vi "Step ADD GND W Parameters.vi"(0 "VISA resource name":refnum<visa-resource-name>, 1 "Scanner Selection in (0)":i32, 2 "Internal scanner?":bool, 5 "GND Test Parameters in":T1={"Current (25 A)"=25.0, "Voltage (8 V)"=8.0, "Hi-Limit (100 mohm)"=100.0, "Lo-Limit (0 mohm)"=0.0, "Dwell (1 s)"=1.0, "Offset (0 mohm)"=0.0, "Auto Offset (OFF)"=FALSE} {"Offset (0 mohm)" format="%#.2f"; "Lo-Limit (0 mohm)" format="%#.2f"; "Hi-Limit (100 mohm)" format="%#.2f"}, 7 "Step Selection (1-200)":i32=1, 9 "Add Step":bool, 11 "error in (no error)":errorcluster) -> (4 "VISA resource name out":refnum<visa-resource-name>, 15 "error out":errorcluster)   [LabVIEW 2014]
doc: "Inserts a GND test with the User defined parameters into the assigned Step Selecton.\n\nIf Add step is set to Edit, it will replace the existing step. If it is set to Add it will insert the new step and increment all steps after the selected step by 1.\n\nSee specifications for Limits."
uses:
  <instrlib>/eec EST 300/eec EST 300.lvlib
  <instrlib>/EEC EST 300/Public/Configure/Steps/Low Level/GND Test Parameters.ctl
panel:
  # "Add"
  # "Edit"
  # "ON"
  # "OFF"
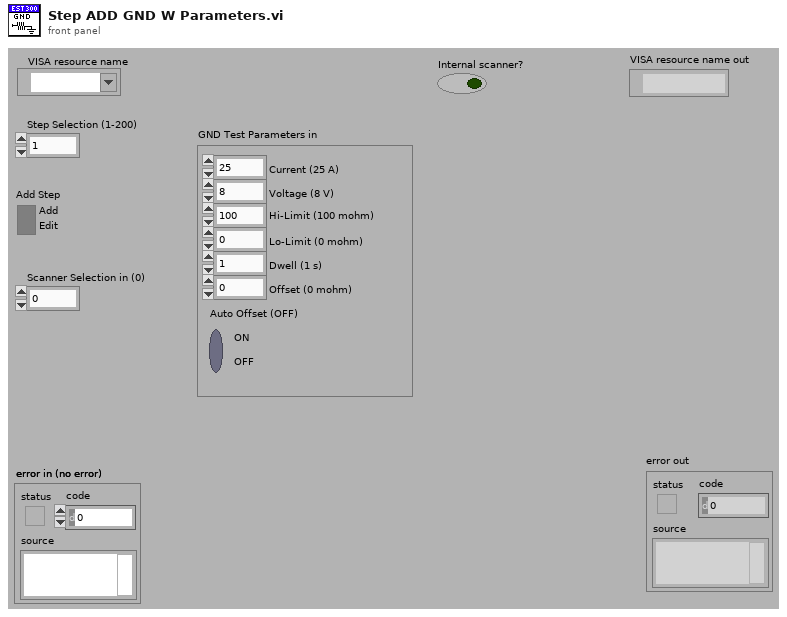
[diagram p1: front panel]
types:
  T1 = typedef "EEC EST 300.lvlib/GND Test Parameters.ctl" = cluster{"Current (25 A)":dbl, "Voltage (8 V)":dbl, "Hi-Limit (100 mohm)":dbl, "Lo-Limit (0 mohm)":dbl, "Dwell (1 s)":dbl, "Offset (0 mohm)":dbl, "Auto Offset (OFF)":bool}
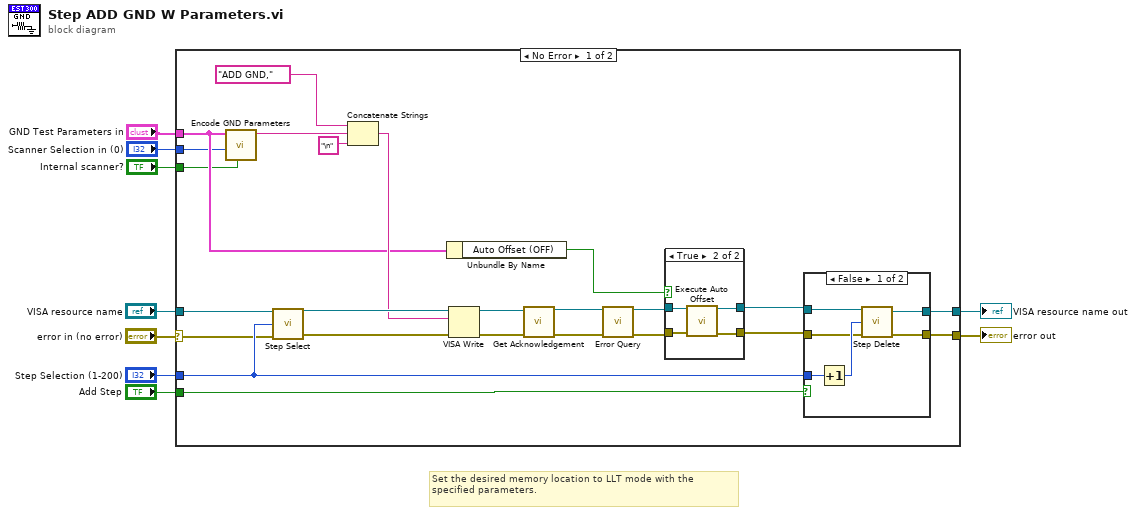
[diagram p0: block diagram]
diagram:
  # "Set the desired memory location to LLT mode with the specified parameters."
  n1 = case shown="No Error" "error in (no error)" {
    selector: "error in (no error)" -> [w22 w49]
    tunnel: [w31 w49] -> w8
    tunnel: [w30 w48] -> w6
    tunnel: "VISA resource name" -> [w23 w48]
    tunnel: "Step Selection (1-200)" -> [w24 _]
    tunnel: "Add Step" -> [w29 _]
    tunnel: "Internal scanner?" -> [w10 _]
    tunnel: "GND Test Parameters in" -> [w12 _]
    tunnel: "Scanner Selection in (0)" -> [w11 _]
    frame No Error {
      n2 = call <instrlib>:"Encode GND Parameters.vi"("scanner? (F:No)"=w10, "Scanner Selection in (0)"=w11, "GND Test Parameters in"=w12) -> ("ADD Parameters out"=w13:string)  [unwired: 6 in, 2 out]
      n3 = call <instrlib>:"Step Select.vi"("VISA resource name"=w23, "Step Number (1)"=w24, "error in (no error)"=w22) -> ("VISA resource name out"=w32:refnum<visa-resource-name>, "error out"=w33:errorcluster)  [unwired: 11 in]
      n4 = Concatenate Strings("ADD GND," ("string"), w13, "\n" ("string")) -> (w27:string)
      n5 = Unbundle By Name(w12) -> ("Auto Offset (OFF)"=w14:bool)
      n6 = VISA Write(VISA resource name=w32, write buffer=w27, error in (no error)=w33) -> (VISA resource name out=w20:refnum<visa-resource-name>, error out=w19:errorcluster)  [unwired: 1 out]
      n7 = call <instrlib>:"Get Acknowledgement.vi"("VISA resource name"=w20, "error in (no error)"=w19) -> ("VISA resource name out"=w26:refnum<visa-resource-name>, "error out"=w25:errorcluster)  [unwired: 12 in]
      n8 = call <instrlib>:"Error Query.vi"("VISA resource name"=w26, "error in (no error)"=w25) -> ("VISA resource name out"=w18:refnum<visa-resource-name>, "error out"=w17:errorcluster)  [unwired: 10 in, 2 out]
      n9 = case shown="True" w14 {
        tunnel: w18 -> [w35 w39]
        tunnel: w17 -> [w34 w36]
        tunnel: [w35 w38] -> w15
        tunnel: [w34 w37] -> w16
        frame False {
        }
        frame True {
          n10 = call <instrlib>:"Execute Auto Offset.vi"("VISA resource name"=w39, "error in (no error)"=w36) -> ("VISA resource name out"=w38:refnum<visa-resource-name>, "error out"=w37:errorcluster)  [unwired: 12 in]
        }
      }
      n11 = case shown="False" w29 {
        tunnel: w24 -> [w45 _]
        tunnel: w16 -> [w43 w46]
        tunnel: w15 -> [w42 w47]
        tunnel: [w41 w46] -> w31
        tunnel: [w40 w47] -> w30
        frame False {
          n12 = Increment(x=w45) -> (x+1=w44:i32)
          n13 = call <instrlib>:"Step Delete.vi"("VISA resource name"=w42, "Step Number (0 = Active Step)"=w44, "error in (no error)"=w43) -> ("VISA resource name out"=w40:refnum<visa-resource-name>, "error out"=w41:errorcluster)  [unwired: 11 in]
        }
        frame True {
        }
      }
    }
    frame Error {
    }
  }
  "error out" <- w8
  "VISA resource name out" <- w6
